vi "Get Bot Angle Using Gyro.vi"(11 "Gyro bias":cluster{"X":dbl, "Y":dbl, "Z":dbl}) -> (2 "GYRO IS FUCKED":bool, 3 "Z Rotation (rads)":dbl)   [LabVIEW 2017]
uses:
  <vilib>/Utility/error.llb/DialogType.ctl
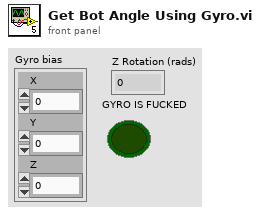
[diagram p1: front panel]
types:
  T1 = typedef "DialogType.ctl" = u16
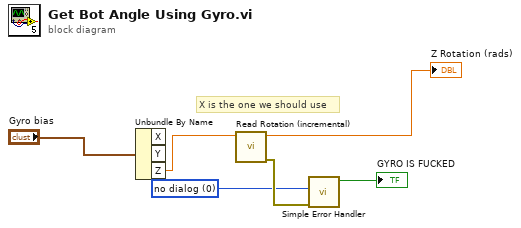
[diagram p0: block diagram]
diagram:
  w3 = T1 0 items=["no dialog", "OK message", "continue or stop message", "OK message + warnings", "continue/stop + warnings"] ("type of dialog (OK msg:1)")
  # "X is the one we should use"
  n1 = Unbundle By Name("Gyro bias") -> ("Z"=w1:dbl)  [unwired: 2 out]
  n2 = call "Read Rotation (incremental).vi"("Gyro Bias"=w1) -> ("error out"=w4:errorcluster, "Z Rotation (rads)"=→"Z Rotation (rads)":dbl)  [unwired: 9 in]
  n3 = call <vilib>:"Simple Error Handler.vi"("type of dialog (OK msg:1)"=w3, "error in (no error)"=w4) -> ("error?"=→"GYRO IS FUCKED":bool)  [unwired: 3 in, 4 out]
